vi "XCAN_W_Vel__R_Crt.vi"() -> ()   [LabVIEW 2016]
uses:
  <vilib>/Stratom, Inc/X-CAN for myRIO (API)/X-CAN Class/Type Definitions/CANFrame.ctl
  <vilib>/Stratom, Inc/X-Modules for myRIO/Type Defs/MXPChannel.ctl
  <vilib>/Stratom, Inc/X-CAN for myRIO (API)/X-CAN Class/Type Definitions/CAN_Speed.ctl
  <vilib>/myRIO/Common/Instrument Driver Framework/myRIO v1.0/UART/vis/myRIO v1.0 Close UART.vi
  <vilib>/myRIO/Common/Instrument Driver Framework/Utilities/vis/FPGA Ref Manager.vi
  <vilib>/myRIO/Common/Instrument Driver Framework/myRIO v1.0/myRIO v1.0 Reset FPGA.vi
  <vilib>/myRIO/Common/Instrument Driver Framework/myRIO v1.0/IRQ/vis/myRIO v1.0 IRQ Info FGV.vi
  <vilib>/myRIO/Common/Instrument Driver Framework/myRIO v1.0/IRQ/vis/myRIO v1.0 Timer IRQ Info FGV.vi
  <vilib>/myRIO/Common/Instrument Driver Framework/myRIO v1.0/IRQ/vis/myRIO v1.0 ISR Agent.vi
  <vilib>/Stratom, Inc/X-CAN for myRIO (API)/X-CAN Class/X-CAN.lvclass
  <vilib>/myRIO/Instrument Drivers/Utilities/Utilities.lvlib
panel:
  out "Data_Gauge":i32(graph)
  out "Raw Data":u8[](array[numeric]) format="%.0x"
  out "Error_Read 3":errorcluster
  out "Numeric":i32
  in  "Set":i32(knob) scale=-7800.0..7800.0
  out "Error_Read 2":errorcluster
  out "CAN Read 2":T1 {"payload" format="%x"; "timestamp" format="%<%I:%M:%S%8u %p\n%x>T"; "identifier" format="%x"}
  out "CAN Read":T1 {"payload" format="%x"; "timestamp" format="%<%I:%M:%S%8u %p\n%x>T"; "identifier" format="%x"}
  in  "stop":bool
  out "Error_Read":errorcluster
  # "Read Current Avg:     0x601    40 D1 30 01 00 00 00 00"
  # "Read Velocity Avg:    0x601    40 D3 30 01 00 00 00 00"
  # "Read Position:            0x601    40 64 60 00 00 00 00 00"
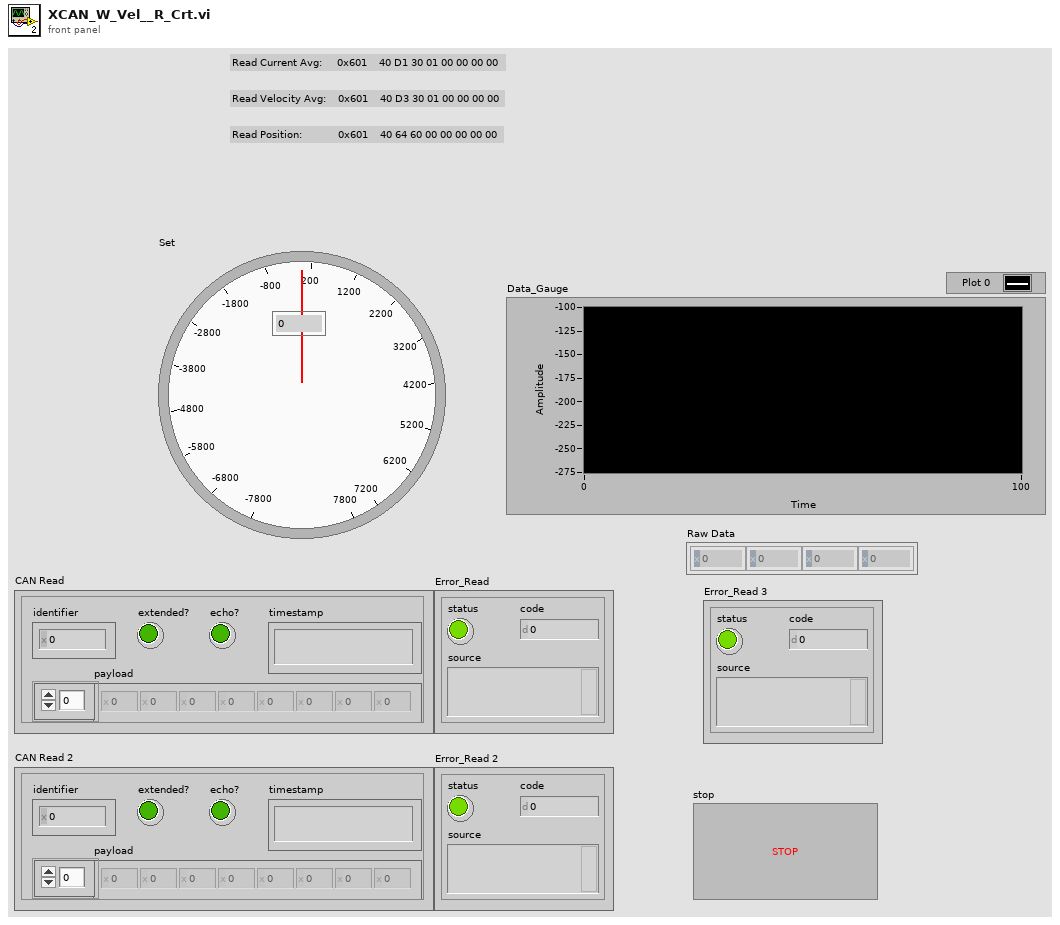
[diagram p1: front panel]
types:
  T1 = typedef "X-CAN.lvclass/CANFrame.ctl" = cluster{"identifier":u32, "extended?":bool, "echo?":bool, "payload":u8[], "timestamp":timestamp}
  T2 = typedef "X-CAN.lvclass/CAN_Speed.ctl" = u8
  T3 = typedef "MXPChannel.ctl" = enum16{"A/MXP", "B/MXP"}
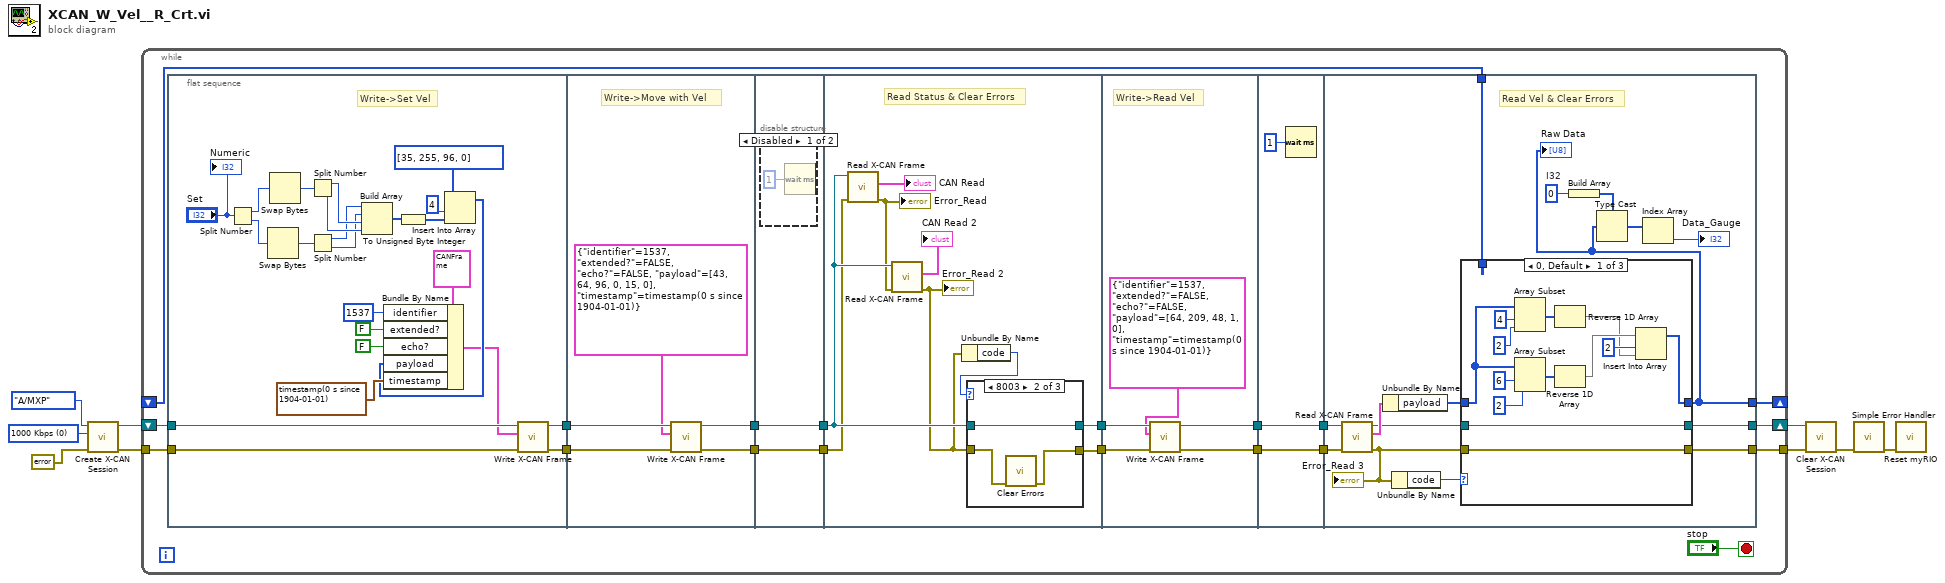
[diagram p0: block diagram]
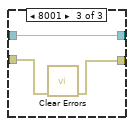
[diagram p4: hidden frame]
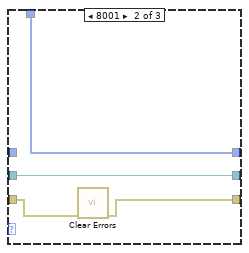
[diagram p5: hidden frame]
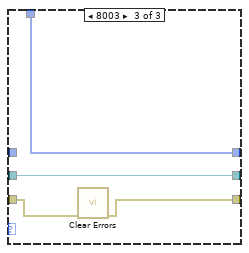
[diagram p6: hidden frame]
diagram:
  w8 = T2 0 items=["125 Kbps"=7, "250 Kbps"=3, "500 Kbps"=1, "1000 Kbps"=0, "95.238 Kbps"=6] ("CAN Speed [Kbps]")
  n1 = call <vilib>:"Create X-CAN Session.vi"("error in (no error)"=errorcluster {"status"=FALSE, "code"=0, "source"=""}, "CAN Speed [Kbps]"=w8, "MXP Channel"=MXPChannel."A/MXP") -> ("error out"=w5:errorcluster, "X-CAN Session out"=w6:refnum<class "X-CAN.lvclass">)  [unwired: 7 in]
  n2 = while {
    tunnel: w5 -> [w23]
    tunnel: [w25] -> w1
    shift-right: [w26] -> w2
    shift-left: w6 -> [w24]
    shift-right: [w11] -> _
    shift-left: _ -> [w10]
    stop <- "stop" stop-if-true
    n3 = flat-sequence {
      tunnel: w24 -> [w52]
      tunnel: w23 -> [w51]
      tunnel: [w50] -> w28
      tunnel: [w49] -> w27
      tunnel: [w57] -> w22
      tunnel: [w56] -> w20
      tunnel: w27 -> [w54]
      tunnel: w28 -> [w55]
      tunnel: w22 -> [w59]
      tunnel: [w59] -> w21
      tunnel: w20 -> [w58]
      tunnel: [w58] -> w19
      tunnel: [w65] -> w17
      tunnel: [w66] -> w16
      tunnel: w19 -> [w62]
      tunnel: w21 -> [w68]
      tunnel: w17 -> [w82]
      tunnel: w16 -> [w81]
      tunnel: [w80] -> w15
      tunnel: [w79] -> w14
      tunnel: w15 -> [w85]
      tunnel: w14 -> [w84]
      tunnel: [w85] -> w13
      tunnel: [w84] -> w12
      tunnel: [w89] -> w25
      tunnel: [w90] -> w26
      tunnel: w12 -> [w91]
      tunnel: w13 -> [w92]
      tunnel: [w88] -> w11
      tunnel: w10 -> [w87]
      frame #0 {
        # "Write->Set Vel"
        n4 = Split Number(x="Set") -> (hi(x)=w42:u16, lo(x)=w41:u16)
        n5 = Swap Bytes(anything=w41) -> (byte swapped=w38:u16)
        n6 = Swap Bytes(anything=w42) -> (byte swapped=w39:u16)
        n7 = Split Number(x=w39) -> (hi(x)=w34:u8, lo(x)=w33:u8)
        n8 = Split Number(x=w38) -> (hi(x)=w32:u8, lo(x)=w31:u8)
        n9 = Build Array(w32, w31, w34, w33) -> (w30:u8[])
        n10 = To Unsigned Byte Integer(number=w30) -> (unsigned 8bit integer=w29:u8[])
        n11 = Insert Into Array(array=u8[] [35, 255, 96, 0], index=4, new element=w29) -> (w36:u8[])
        n12 = Bundle By Name(cluster=T1 {"identifier"=0, "extended?"=FALSE, "echo?"=FALSE, "payload"=[], "timestamp"=timestamp(0 s since 1904-01-01)} ("CAN Frame"), "identifier"=u32 1537, "extended?"=FALSE, "echo?"=FALSE, "payload"=w36, "timestamp"=timestamp(0 s since 1904-01-01)) -> (w35:T1)
        n13 = call <vilib>:"Write X-CAN Frame.vi"("error in"=w51, "CAN Frame"=w35, "X-CAN Session in"=w52) -> ("error out"=w49:errorcluster, "X-CAN Session out"=w50:refnum<class "X-CAN.lvclass">)  [unwired: 7 in]
        "Numeric" <- "Set"
      }
      frame #1 {
        # "Write->Move with Vel"
        n14 = call <vilib>:"Write X-CAN Frame.vi"("error in"=w54, "CAN Frame"=T1 {"identifier"=1537, "extended?"=FALSE, "echo?"=FALSE, "payload"=[43, 64, 96, 0, 15, 0], "timestamp"=timestamp(0 s since 1904-01-01)} ("CAN Write 2"), "X-CAN Session in"=w55) -> ("error out"=w56:errorcluster, "X-CAN Session out"=w57:refnum<class "X-CAN.lvclass">)  [unwired: 7 in]
      }
      frame #2 {
        n15 = disable-structure shown="Disabled" {
          frame Disabled {
            n16 = Wait (ms)(milliseconds to wait=u32 1) -> ()  [unwired: 1 out]
          }
          frame Enabled {
          }
        }
      }
      frame #3 {
        # "Read Status & Clear Errors"
        n17 = call <vilib>:"Read X-CAN Frame.vi"("error in"=w62, "X-CAN Session in"=w68) -> ("error out"=w61:errorcluster, "CAN Frame"=→"CAN Read":T1)  [unwired: 7 in, 1 out]
        "Error_Read" <- w61
        n18 = call <vilib>:"Read X-CAN Frame.vi"("error in"=w61, "X-CAN Session in"=w68) -> ("error out"=w67:errorcluster, "CAN Frame"=→"CAN Read 2":T1)  [unwired: 7 in, 1 out]
        "Error_Read 2" <- w67
        n19 = Unbundle By Name(w67) -> ("code"=w69:i32)
        n20 = case shown="8003" w69 {
          tunnel: w68 -> [w71 w72 w75]
          tunnel: w67 -> [w70 w74 w77]
          tunnel: [w70 w73 w76] -> w66
          tunnel: [w71 w72 w75] -> w65
          frame 0, Default {
          }
          frame 8003 {
            n21 = call <vilib>:"Clear Errors.vi"("error in (no error)"=w74) -> ("error out"=w73:errorcluster)  [unwired: 5 in, 1 out]
          }
          frame 8001 {
            n22 = call <vilib>:"Clear Errors.vi"("error in (no error)"=w77) -> ("error out"=w76:errorcluster)  [unwired: 5 in, 1 out]
          }
        }
      }
      frame #4 {
        # "Write->Read Vel"
        n23 = call <vilib>:"Write X-CAN Frame.vi"("error in"=w81, "CAN Frame"=T1 {"identifier"=1537, "extended?"=FALSE, "echo?"=FALSE, "payload"=[64, 209, 48, 1, 0], "timestamp"=timestamp(0 s since 1904-01-01)} ("CAN Write"), "X-CAN Session in"=w82) -> ("error out"=w79:errorcluster, "X-CAN Session out"=w80:refnum<class "X-CAN.lvclass">)  [unwired: 7 in]
      }
      frame #5 {
        n24 = Wait (ms)(milliseconds to wait=u32 1) -> ()  [unwired: 1 out]
      }
      frame #6 {
        w94 = 0  # I32
        # "Read Vel & Clear Errors"
        n25 = call <vilib>:"Read X-CAN Frame.vi"("error in"=w91, "X-CAN Session in"=w92) -> ("error out"=w98:errorcluster, "CAN Frame"=w100:T1, "X-CAN Session out"=w99:refnum<class "X-CAN.lvclass">)  [unwired: 7 in]
        "Error_Read 3" <- w98
        n26 = Unbundle By Name(w100) -> ("payload"=w97:u8[])
        n27 = Unbundle By Name(w98) -> ("code"=w96:i32)
        n28 = case shown="0, Default" w96 {
          tunnel: w99 -> [w112 w117 w121]
          tunnel: w98 -> [w113 w115 w119]
          tunnel: w97 -> [w105 _ _]
          tunnel: [w112 w117 w121] -> w90
          tunnel: [w113 w114 w118] -> w89
          tunnel: [w103 w116 w120] -> w88
          tunnel: w87 -> [_ w116 w120]
          frame 0, Default {
            n29 = Array Subset(array=w105, index=4, length=2) -> (w109:u8[])
            n30 = Array Subset(array=w105, index=6, length=2) -> (w108:u8[])
            n31 = Reverse 1D Array(array=w109) -> (reversed array=w101:u8[])
            n32 = Reverse 1D Array(array=w108) -> (reversed array=w102:u8[])
            n33 = Insert Into Array(array=w102, index=2, new element=w101) -> (w103:u8[])
          }
          frame 8001 {
            n34 = call <vilib>:"Clear Errors.vi"("error in (no error)"=w115) -> ("error out"=w114:errorcluster)  [unwired: 5 in, 1 out]
          }
          frame 8003 {
            n35 = call <vilib>:"Clear Errors.vi"("error in (no error)"=w119) -> ("error out"=w118:errorcluster)  [unwired: 5 in, 1 out]
          }
        }
        "Raw Data" <- w88
        n36 = Build Array(w94) -> (w95:i32[])
        n37 = Type Cast(type=w95, x=w88) -> (*(type *) &x=w93:i32[])
        n38 = Index Array(array=w93) -> (element=→"Data_Gauge":i32)  [unwired: 1 in]
      }
    }
  }
  n39 = call <vilib>:"Clear X-CAN Session.vi"("error in (no error)"=w1, "X-CAN Session in"=w2) -> ("error out"=w4:errorcluster)  [unwired: 9 in]
  n40 = call <vilib>:"Simple Error Handler.vi"("error in (no error)"=w4) -> ("error out"=w3:errorcluster)  [unwired: 4 in, 4 out]
  n41 = call <vilib>:"Reset myRIO.vi"("error in (no error)"=w3) -> ()  [unwired: 10 in, 1 out]
